vi "Get ErrorMessage.vi"(8 "error in (no error)":errorcluster, 11 "Error Code":i32) -> (0 "error out":errorcluster, 2 "Error Message":string, 3 "Error Code":i32)   [LabVIEW 2021, in "EventManagerLibrary.lvlib" / "EventManagerErrors.lvclass"]
uses:
  EventManagerErrors.lvclass
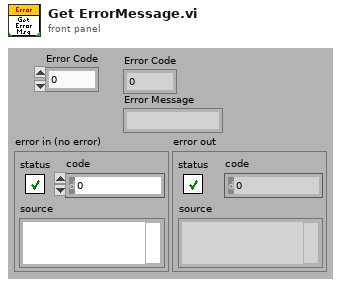
[diagram p1: front panel]
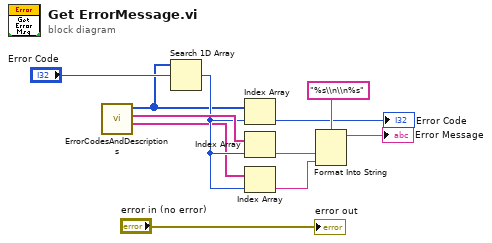
[diagram p0: block diagram]
diagram:
  n1 = call "ErrorCodesAndDescriptions.vi"() -> ("Error Descriptions"=w5:string[], "Error Names"=w10:string[], "Error Codes"=w6:i32[])  [unwired: 9 in]
  n2 = Search 1D Array(1D array=w6, element="Error Code") -> (index of element=w9:i32)  [unwired: 1 out]
  n3 = Index Array(array=w6, index=w9) -> (element=→"Error Code":i32)
  n4 = Index Array(array=w10, index=w9) -> (element=w8:string)
  n5 = Index Array(array=w5, index=w9) -> (element=w7:string)
  n6 = Format Into String(format string="%s\\n\\n%s", w8, w7) -> (resulting string=→"Error Message":string)  [unwired: 2 in, 1 out]
  "error out" <- "error in (no error)"
